vi "Write Phase (0-1).vi"(8 "error in (no error)":errorcluster, 10 "Phase (0-1)":dbl, 11 "SAM in":refnum<class "SAM.lvclass">) -> (0 "error out":errorcluster, 3 "SAM out":refnum<class "SAM.lvclass">)   [LabVIEW 2020, in "SAM.lvclass"]
uses:
  SAM.lvclass
  SAM.lvclass/SAM.ctl
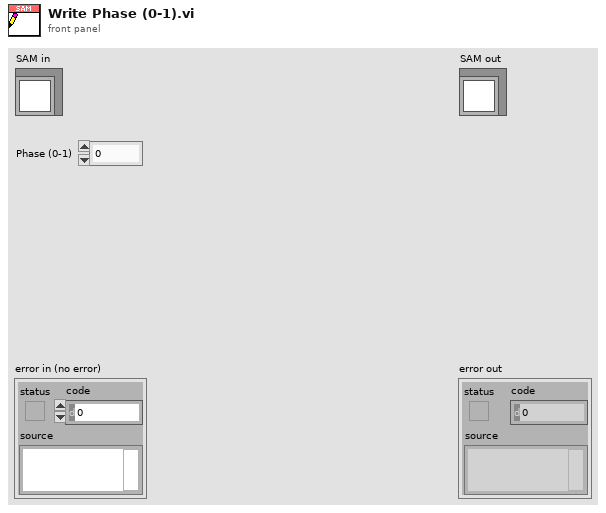
[diagram p1: front panel]
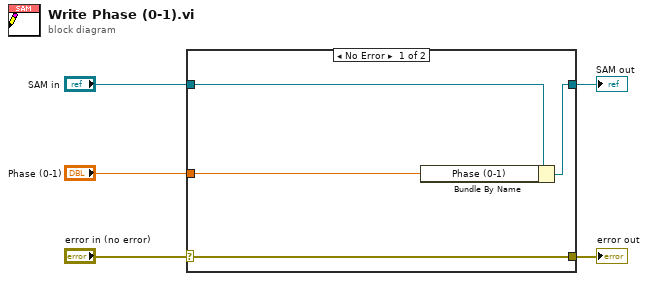
[diagram p0: block diagram]
diagram:
  n1 = case shown="No Error" "error in (no error)" {
    selector: "error in (no error)" -> [w9 w10]
    tunnel: [w9 w10] -> w4
    tunnel: [w7 w11] -> w2
    tunnel: "SAM in" -> [w8 w11]
    tunnel: "Phase (0-1)" -> [w6 _]
    frame No Error {
      n2 = Bundle By Name(cluster=w8, "Phase (0-1)"=w6) -> (w7:refnum<class "SAM.lvclass">)
    }
    frame Error {
    }
  }
  "error out" <- w4
  "SAM out" <- w2
